vi "PSUTI_Queue Name Utility.vi"() -> (2 "Queue Names":T1)   [LabVIEW 2016]
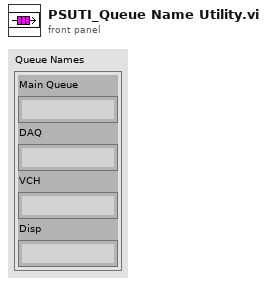
[diagram p1: front panel]
types:
  T1 = cluster{"Main Queue":string, "DAQ":string, "VCH":string, "Disp":string}
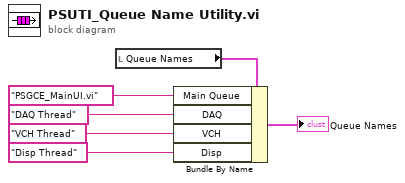
[diagram p0: block diagram]
diagram:
  n1 = local read "Queue Names"() -> (w6:T1)
  n2 = Bundle By Name(cluster=w6, "Main Queue"="PSGCE_MainUI.vi" ("Name"), "DAQ"="DAQ Thread", "VCH"="VCH Thread" ("DAQ"), "Disp"="Disp Thread" ("DAQ")) -> (→"Queue Names":T1)
